vi "Scope_Fast_PID.vi"() -> ()   [LabVIEW 2013]
uses:
  <vilib>/userdefined/High Color/nirio_resource_hc.ctl
  FPGA/DataMode.ctl
  <vilib>/Analysis/4window.llb/windowTd.ctl
  Host/Scope/controls/power_spectrum_unit.ctl
  Host/Scope5782/Scope/controls/5782_trigger_type.ctl
  Host/Scope/controls/Data_calc_mode.ctl
  Host/Scope/controls/Data_display_mode.ctl
  Host/Scope/controls/Graph_references.ctl
  Host/Scope/controls/graph_controls.ctl
  Host/Scope/controls/Channel_select.ctl
  Host/Communication/response.ctl
  Host/Communication/driver_status.ctl
  Host/Communication/Driver/RemoteConnection/RemoteReferences.ctl
  Host/Scope5782/Config/FPGAref_5782.ctl
  Host/Communication/Driver/TcpServerDriver/TcpServerDriver.lvclass
  Host/Scope5782/Scope/controls/c_t_type.ctl
  Host/Scope/controls/ScopeMode.ctl
  FPGA/fpga_settings.ctl
  Host/Scope5782/Scope/controls/Memory block.ctl
  Host/Communication/global_stop.vi
  <vilib>/FPGAPlugInAG/PXIe-7975R/niLvFpga_Open_PXIe-7975R.vi
  <vilib>/rvi/interface/common/dynamic/niFpgaDynamicAddResources.vi
  <vilib>/rvi/interface/common/niFpgaWaitOnOcc.vi
  <vilib>/Utility/error.llb/Error Cluster From Error Code.vi
  <vilib>/rvi/errors/niLvFpgaAdjustHostInterfaceError.vi
  <vilib>/FPGAPlugInAG/Dynamic/niLvFpga_Close_Dynamic.vi
  <vilib>/rvi/interface/nirviOpenFPGA/nirviOpenFPGA.xnode
  FPGA Bitfiles/FPGAmain_5782_Fast_PID_eL07vsNfjYY.lvbitx
  <vilib>/rvi/interface/nirviReadWriteControl/nirviReadWriteControl.xnode
  <vilib>/rvi/FXPMathLib/FxpInterpret/XNode/nifxpmath_Interpret.xnode
  <vilib>/rvi/interface/nirviMethod/nirviMethod.xnode
  <vilib>/rvi/interface/nirviCloseFPGA/nirviCloseFPGA.xnode
  Host/Utilities/Ticker/Ticker.lvclass
  NiFpgaLv.dll
  <vilib>/rvi/interface/Simulation/niFpgaSimulationCallBeginRW.vi
  Host/Communication/Driver/RemoteConnection/RemoteConnection.lvclass
  <vilib>/FPGAPlugInAG/Dynamic/niLvFpga_WriteFifo_Dynamic.vi
  <vilib>/rvi/errors/niLvFpgaMergeErrorWithErrorCode.vi
  <vilib>/Analysis/NI_AALPro.lvlib
panel:
  in  "Acquire samples":u16
  in  "Trigger delay":u16
  in  "Feedback delay":u16
  in  "Beam/FF enabled":bool
  in  "Setpoint enabled":bool
  in  "show feedforward":bool
  in  "show beam":bool
  in  "show setpoint":bool
  in  "Feed forward":path
  in  "Beam":path
  in  "Setpoint":path
  in  "High speed transfer to host":bool=TRUE
  in  "Output enabled":bool=TRUE
  in  "ch1 DC offset":dbl caption="DC offset\nChannel 1"
  in  "ch0 DC offset":dbl caption="DC offset\nChannel 0"
  in  "Output delay delta":dbl(slide) scale=0.0..6.0
  in  "Output delay":dbl(slide) scale=0.0..6.0
  in  "Output mixer fequency [MHz]":dbl
  in  "Trigger":T1
  in  "Mode":T2
  in  "Mixer freq [MHz]":dbl
  in  "unwrap phase":bool
  in  "Kp AM":fxp<+/-,32,4> caption="Kp"
  in  "Kd/T AM":fxp<+/-,32,4> caption="Kd/T"
  in  "Ki*T AM":fxp<+/-,32,4> caption="Ki*T"
  in  "Feedback AM":bool caption="Feedback"
  in  "Kp":fxp<+/-,32,4>
  in  "Kd/T":fxp<+/-,32,4>
  in  "Ki*T":fxp<+/-,32,4>
  in  "Feedback":bool
  in  "c(t) AM":bool
  in  "c(t) phase":bool
  in  "b":fxp<+/-,16,2>
  in  "a":fxp<+/-,16,2>
  in  "Fequency [kHz]":dbl format="%#_8g"
  in  "#bins":i32=1 min=1 max=16
  in  "Unit":T3
  in  "Window":T4=1 items=["Rectangle"=0, "Hanning"=1, "Hamming"=2, "Blackman-Harris"=3, "Exact Blackman"=4, "Blackman"=5, "Flat Top"=6, "4 Term B-Harris "=7, "7 Term B-Harris"=8, "Low Sidelobe"=9, "Blackman Nuttall"=11, "Triangle"=30, "Bartlett-Hanning"=31, "Bohman"=32, "Parzen"=33, "Welch"=34, "Kaiser"=60, "Dolph-Chebyshev"=61, "Gaussian"=62]
  in  "Chart length":i32=400000
  in  "Trigmode":enum32{"Triggered", "Continuous"}(radio)
  in  "Refence for phase":T5
  in  "Graph_refs":T6
  out "Lower chart":dbl[][](graph)
  out "Upper chart":dbl[][](graph)
  out "Lower graph":i16[][](graph)
  in  "Buffer":T8
  in  "Display":T9
  in  "Ch1 Q":bool
  in  "Ch1 I":bool
  in  "Ch0 Q":bool
  in  "Ch0 I":bool
  in  "Ch1":bool
  in  "Ch0":bool
  out "stop 2":bool
  in  "Zoom freq X":bool
  in  "Zoom freq Y":bool
  in  "Zoom time Y":bool
  in  "Zoom time X":bool
  in  "Samples per 5782 record":i32
  in  "Phase offset (deg)":dbl
  in  "Fequency [MHz]":dbl format="%#_8g"
  out "freqdata":cluster{"f0":dbl, "df":dbl, "magnitude":dbl[]}[](graph)
  out "Upper graph":i16[][](graph)
  in  "Rumode":bool
  in  "Singleshot":bool
  out "error IO":errorcluster
  in  "stop":bool
  in  "resource name":T10="PXI1Slot18"
  out "Clocking Option Configured?":bool
  out "Configured?":bool
  # "Auto Zoom"
  # "5782"
  # "Delays"
  # "FFT"
  # "Auto Zoom"
  # "FPGA setup"
  # "V"
  # "V"
  # "ns"
  # "Output delay"
  # "ps"
  # "Output delay delta"
  # "Amplitude"
  # "Phase"
  # "Amplitude modulation"
  # "Simulated data"
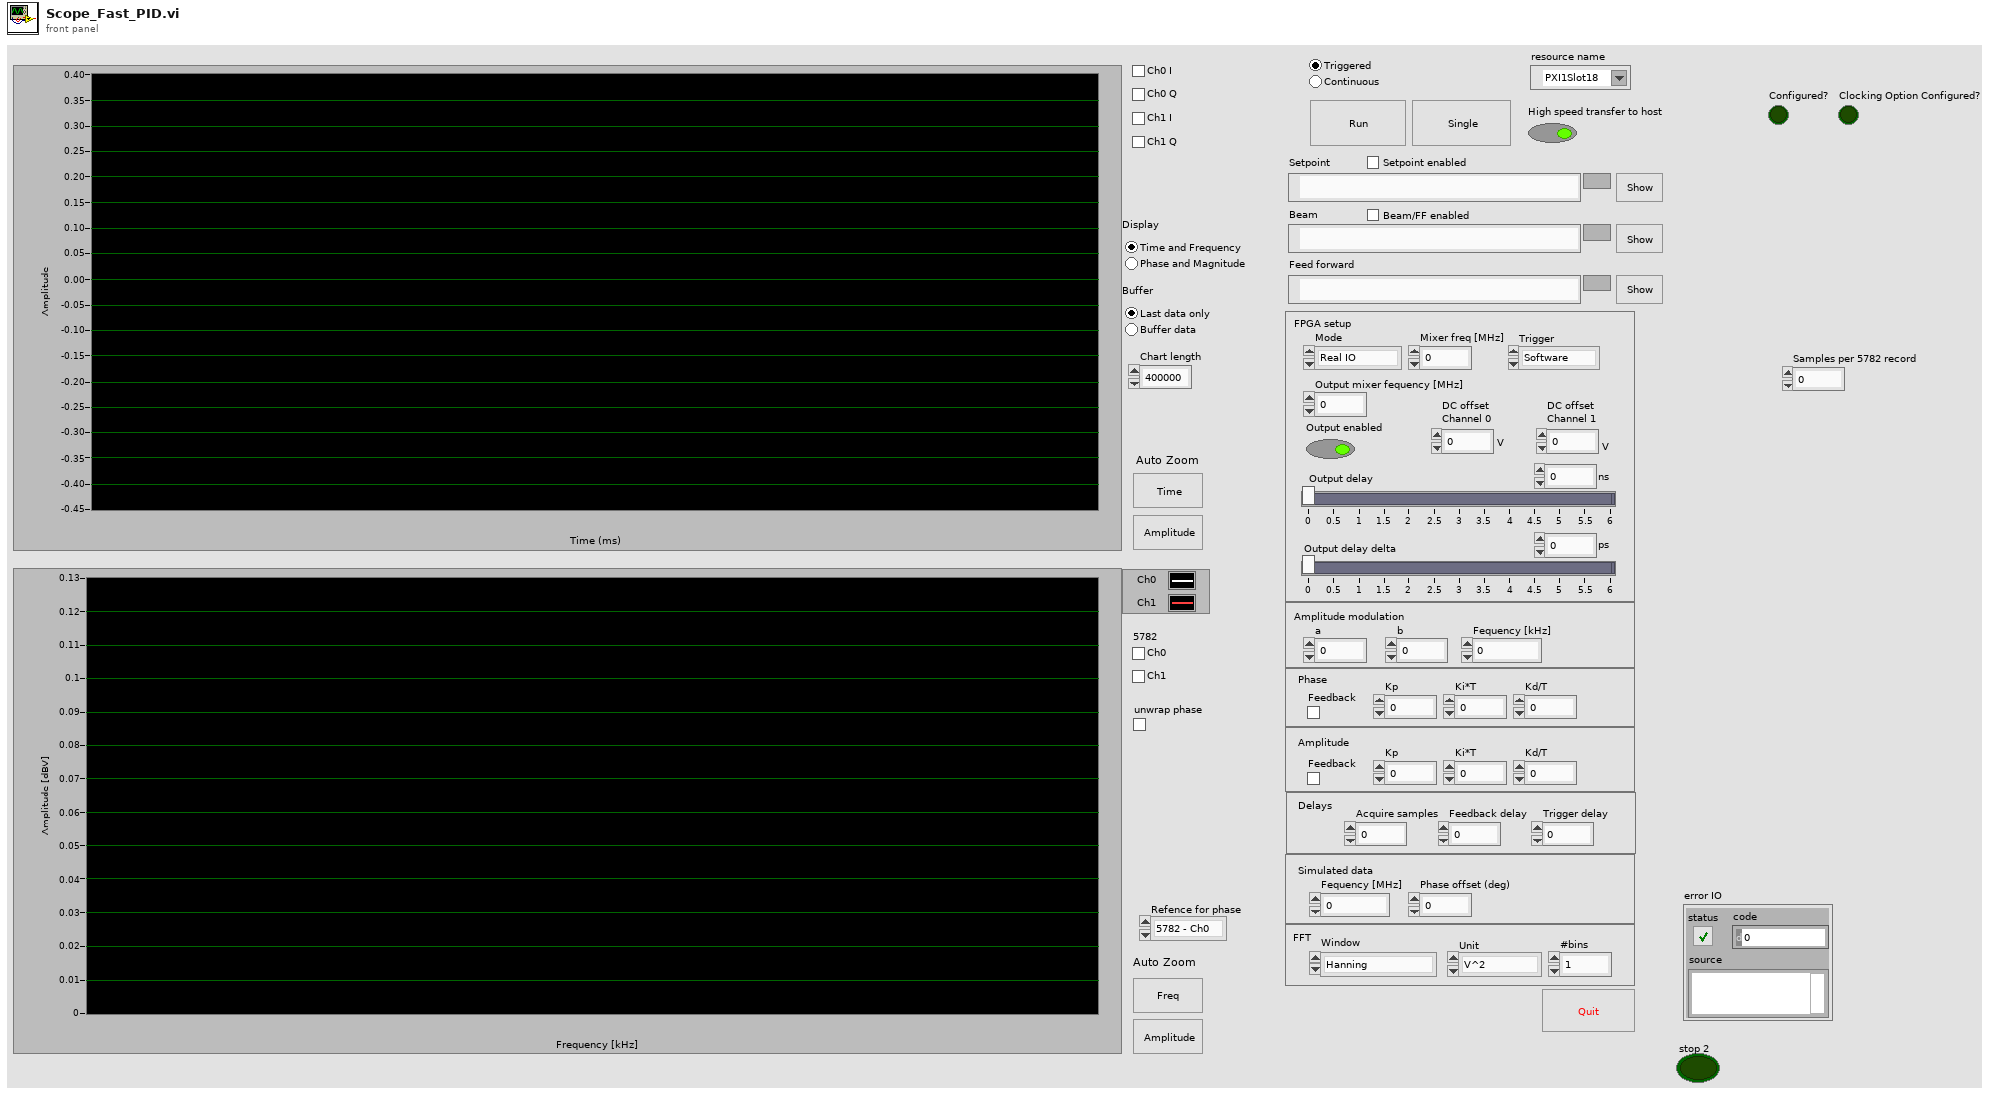
[diagram p1: front panel]
types:
  T1 = typedef "5782_trigger_type.ctl" = enum16{"Software", "Trigger input"}
  T2 = typedef "DataMode.ctl" = enum16{"Real IO", "Simulated"}
  T3 = typedef "power_spectrum_unit.ctl" = enum16{"V^2", "V", "dBV"}
  T4 = typedef "NI_AALPro.lvlib/windowTd.ctl" = u32
  T5 = typedef "Channel_select.ctl" = enum16{"5782 - Ch0", "5782 - Ch1"}
  T6 = typedef "Graph_references.ctl" = cluster{"upper":T7, "lower":T7, "Freq graph":refnum<vi>}
  T7 = typedef "graph_controls.ctl" = cluster{"Graph":refnum<vi>, "Time btn":refnum<vi>, "Amplitude btn":refnum<vi>, "Chart":refnum<vi>}
  T8 = typedef "Data_display_mode.ctl" = enum32{"Last data only", "Buffer data"}
  T9 = typedef "Data_calc_mode.ctl" = enum32{"Time and Frequency", "Phase and Magnitude"}
  T10 = typedef "nirio_resource_hc.ctl" = tag
  T11 = typedef "FPGAref_5782.ctl" = refnum<k20>
  T12 = typedef "RemoteConnection.lvclass/RemoteReferences.ctl" = cluster{"a":refnum<vi>, "b":refnum<vi>, "fm":refnum<vi>, "Output delay":refnum<vi>, "Output delay delta":refnum<vi>}
  T13 = typedef "response.ctl" = cluster{"driver status":T14, "Sender":string, "Type":i32, "Variant":variant}
  T14 = typedef "driver_status.ctl" = enum16{"Normal", "Startup", "Connection lost", "Reconnected", "Timeout", "Idle", "Busy"}
  T15 = enum8{"Internal Clock PLL Off", "Internal Clock PLL On (REF IN)", "External Clock (CLK_IN)", "Internal Clock PLL On (IoModSyncClk)"}
  T16 = typedef "message_queue.ctl" = refnum<queue>
  T17 = typedef "scope_params_5782.ctl" = cluster{"scope mode":T18, "ticker":refnum<class "Ticker.lvclass">, "samples per record":i32, "FPGA ref":T11, "data mode":T2, "5782 Trigger":T1, "Chart length":i32, "RemoteConnection":refnum<class "RemoteConnection.lvclass">, "last phase":dbl[], "Feedforward":T19}
  T18 = typedef "ScopeMode.ctl" = enum16{"Stopped", "Single", "Running", "Continuous"}
  T19 = typedef "Feedforward.ctl" = cluster{"Beam I":dbl[], "Beam Q":dbl[], "Feedforward I":dbl[], "Feedforward Q":dbl[], "Setpoint I":dbl[], "Setpoint Q":dbl[]}
  T20 = typedef "c_t_type.ctl" = enum16{"Phase", "AM", "Both", "None"}
  T21 = typedef "fpga_settings.ctl" = enum16{"Feedback Enable", "New FIR coeffs", "FIR shift", "Enable filter", "Set Downsample", "Downsample", "CIC Gain", "Record length", "Trigger samples", "Quiet time", "a_am", "b_am", "Use fixed delay", "fixed sin_fi", "fixed cos_fi", "Ki*Tau", "Kp", "Kd_Tau", "Fi_start", "Fi_delta", "DC_offs 0", "DC_offs 1", "DC_offs 2", "DC_offs 3", "Ki*Tau am", "Kp am", "Kd_Tau am", "Feedback AM", "Trigger delay", "Feedback delay", "Setpoint enable", "Beam enable", "Samples to acquire"}
  T22 = typedef "Memory block.ctl" = enum16{"Setpoint", "Beam"}
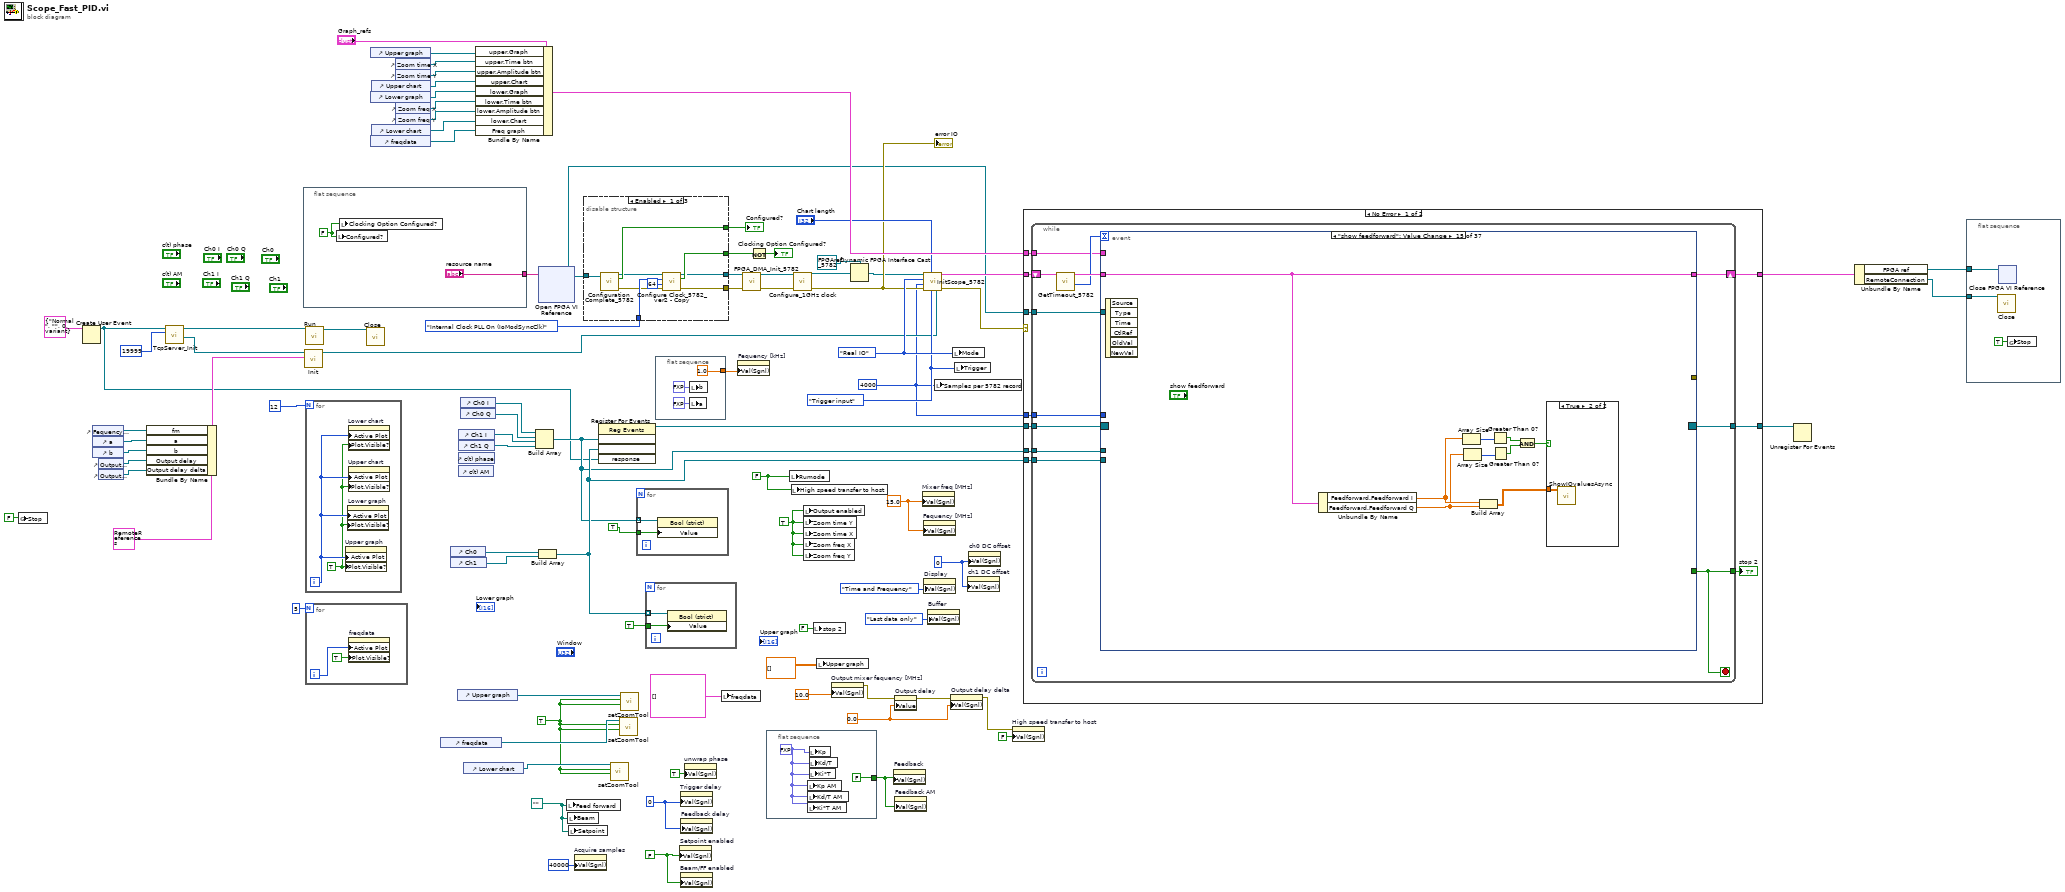
[diagram p0: block diagram]
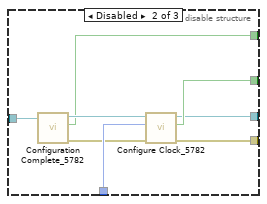
[diagram p2: hidden frame]
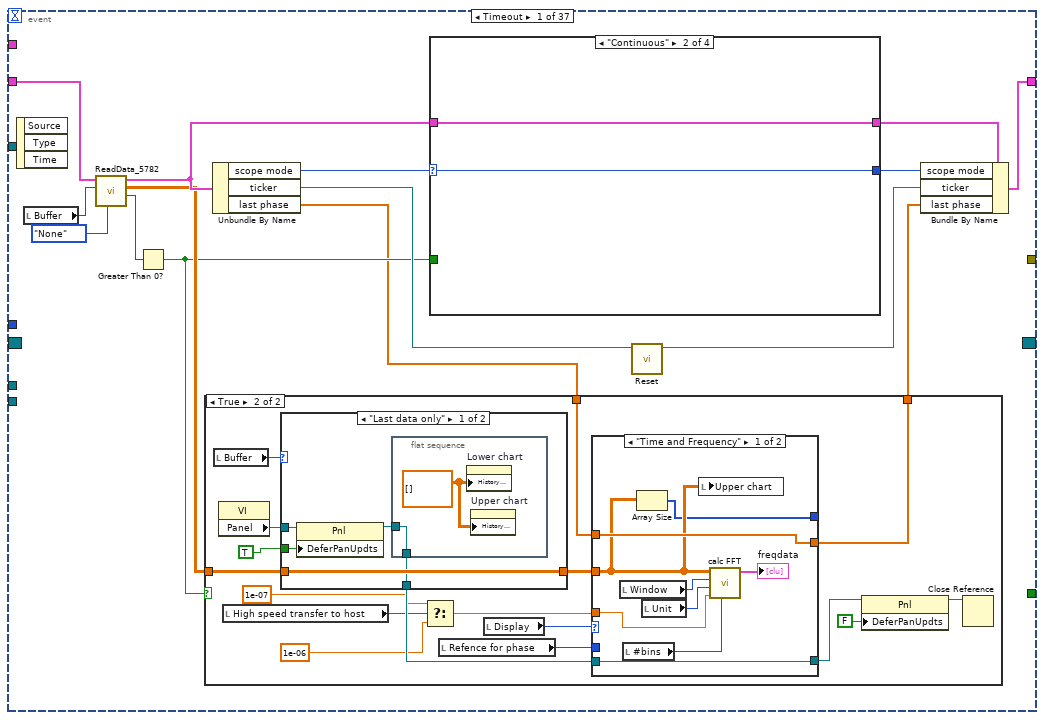
[diagram p4: hidden frame]
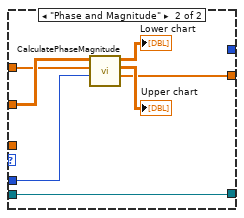
[diagram p7: hidden frame]
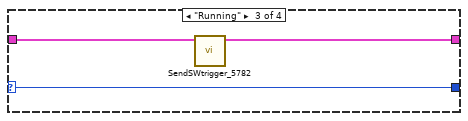
[diagram p9: hidden frame]
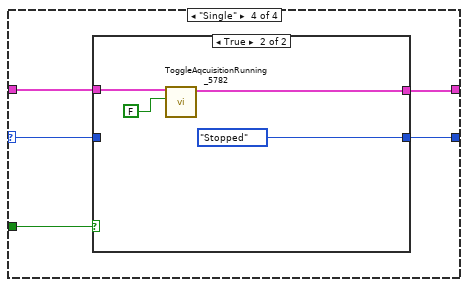
[diagram p10: hidden frame]
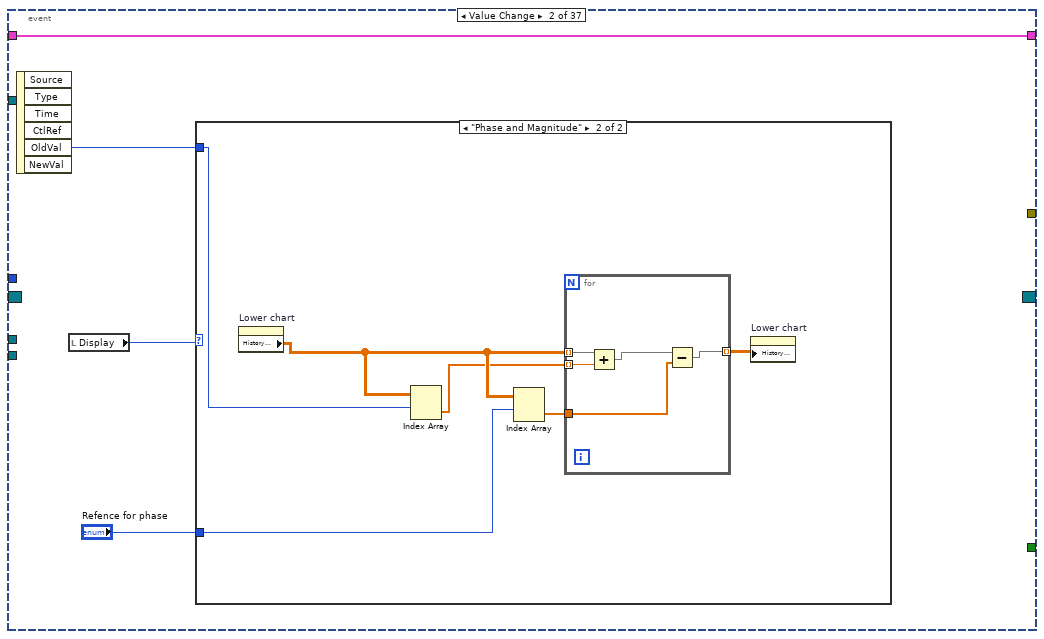
[diagram p12: hidden frame]
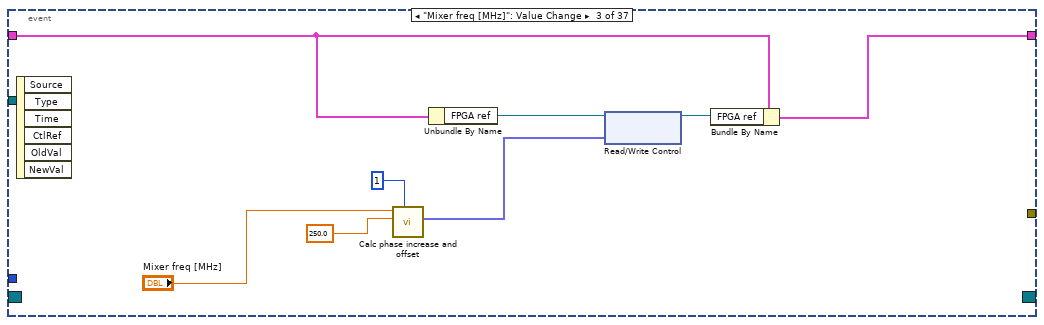
[diagram p14: hidden frame]
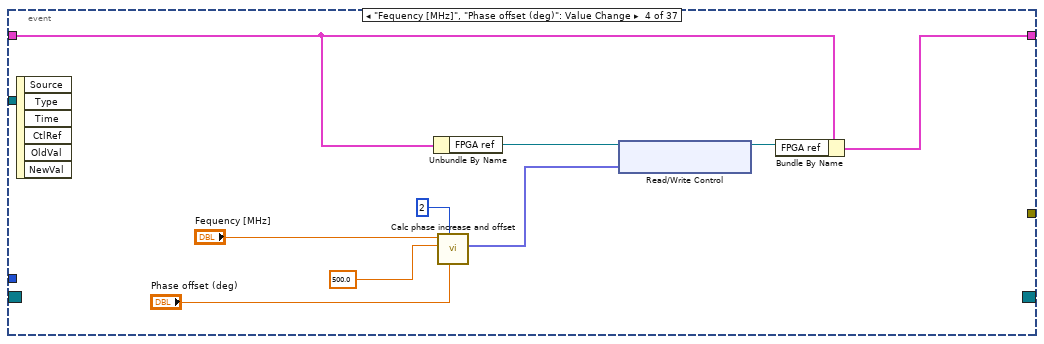
[diagram p15: hidden frame]
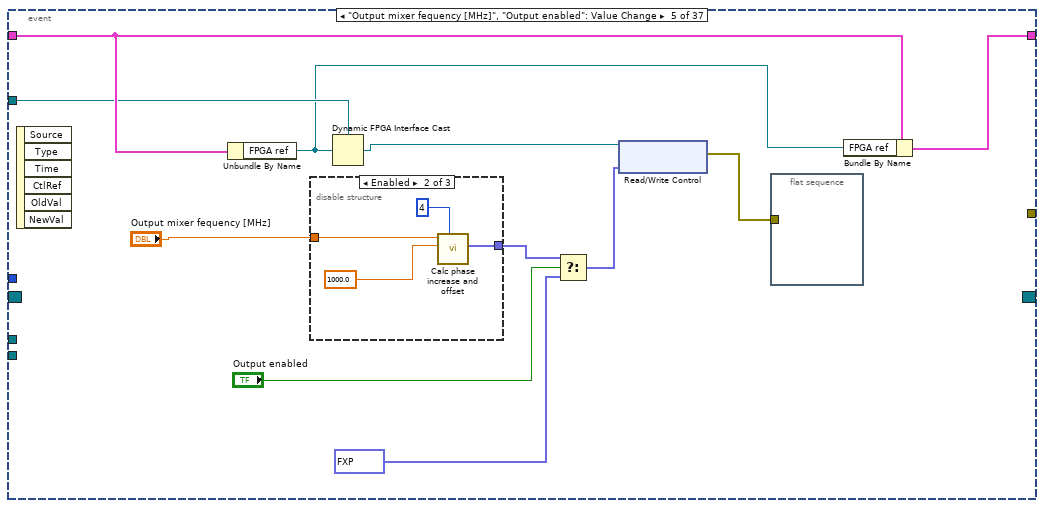
[diagram p16: hidden frame]
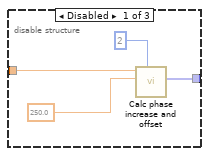
[diagram p17: hidden frame]
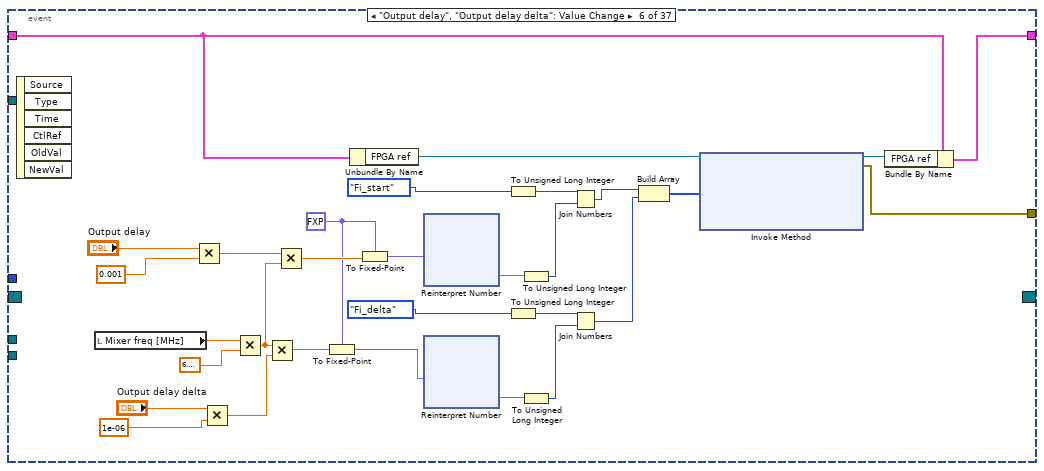
[diagram p19: hidden frame]
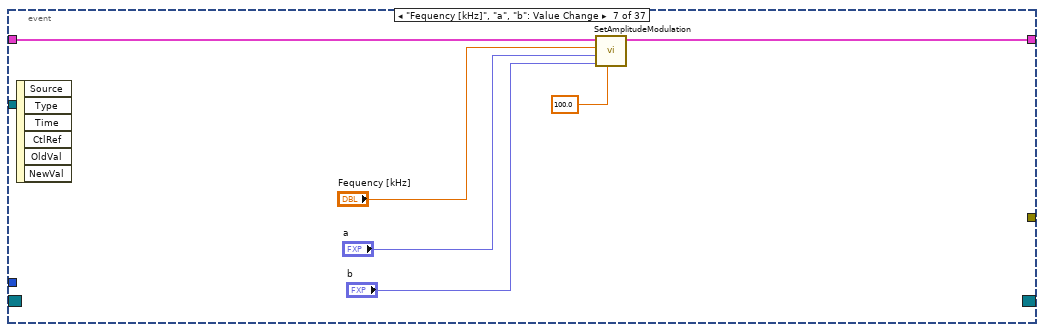
[diagram p20: hidden frame]
diagram:
  w2 = path "" ("Feed forward")
  w3 = FALSE ("Value (Signaling)")
  w4 = u16 0 ("Value (Signaling)")
  w40 = i16 0 ("Value (Signaling)")
  w41 = 0.0 ("Value (Signaling)")
  w63 = 5782_trigger_type."Trigger input" ("Trigger")
  w22 = TRUE ("Zoom  X")
  w15 = TRUE ("Rumode")
  w75 = DataMode."Real IO" ("Mode")
  w8 = 4000 ("Samples to aqcuire")
  w7 = FALSE ("Rumode")
  w85 = 15.0 ("Mixer requency [MHz]")
  n1 = global write "global_stop.vi" "Stop"(FALSE ("Stop")) -> ()
  n2 = Create User Event(user event datatype=T13 {"driver status"=enum."Normal", "Sender"="", "Type"=0, "Variant"=variant} ("response")) -> (user event=w28:refnum<user-event>)  [unwired: 1 in, 1 out]
  n3 = control-ref of="Fequency [kHz]"() -> (w30:refnum<vi>)
  n4 = control-ref of="a"() -> (w31:refnum<vi>)
  n5 = control-ref of="b"() -> (w29:refnum<vi>)
  n6 = control-ref of="Output delay"() -> (w18:refnum<vi>)
  n7 = control-ref of="Output delay delta"() -> (w17:refnum<vi>)
  n8 = Bundle By Name(cluster=T12 {"a"=refnum, "b"=refnum, "fm"=refnum, "Output delay"=refnum, "Output delay delta"=refnum} ("refs"), "fm"=w30, "a"=w31, "b"=w29, "Output delay"=w18, "Output delay delta"=w17) -> (w38:T12)
  n9 = call "TcpServer_Init.vi"("local port"=u16 19999, "response event"=w28) -> ("Message queue"=w36:T16, "TcpServerDriver"=w33:refnum<class "TcpServerDriver.lvclass">)  [unwired: 8 in]
  n10 = flat-sequence {
    tunnel: ["resource name"] -> w76
    frame #0 {
      w90 = FALSE ("Trigger Acquisition")
      n11 = local write "Configured?"(w90) -> ()
      n12 = local write "Clocking Option Configured?"(w90) -> ()
    }
  }
  n13 = call "Init.vi"("refs"=w38, "server queue"=w36) -> ("RemoteConnection"=w27:refnum<class "RemoteConnection.lvclass">)  [unwired: 9 in]
  n14 = for {
    N: 12 -> [_]
    i -> [w93]
    w92 = TRUE ("Plot.Visible")
    n15 = property on="Upper graph" class="WFGraph (strict)"("Active Plot"=w93, "Plot.Visible?"=w92) -> ()  [unwired: 2 in, 2 out]
    n16 = property on="Lower graph" class="WFGraph (strict)"("Active Plot"=w93, "Plot.Visible?"=w92) -> ()  [unwired: 2 in, 2 out]
    n17 = property on="Lower chart" class="WFChart (strict)"("Active Plot"=w93, "Plot.Visible?"=w92) -> ()  [unwired: 2 in, 2 out]
    n18 = property on="Upper chart" class="WFChart (strict)"("Active Plot"=w93, "Plot.Visible?"=w92) -> ()  [unwired: 2 in, 2 out]
  }
  n19 = for {
    N: 5 -> [_]
    i -> [w94]
    n20 = property on="freqdata" class="WFGraph (strict)"("Active Plot"=w94, "Plot.Visible?"=TRUE ("Plot.Visible")) -> ()  [unwired: 2 in, 2 out]
  }
  n21 = call-dynamic "Run.vi"("BaseDriver in"=w33) -> ("BaseDriver out"=w34:refnum<class "TcpServerDriver.lvclass">)  [unwired: 9 in, 1 out]
  n22 = call-dynamic "Close.vi"("BaseDriver in"=w34) -> ()  [unwired: 9 in, 2 out]
  n23 = control-ref of="Upper graph"() -> (w60:refnum<vi>)
  n24 = control-ref of="Lower graph"() -> (w56:refnum<vi>)
  n25 = control-ref of="freqdata"() -> (w52:refnum<vi>)
  n26 = control-ref of="Upper chart"() -> (w57:refnum<vi>)
  n27 = control-ref of="Lower chart"() -> (w53:refnum<vi>)
  n28 = control-ref of="Zoom time X"() -> (w59:refnum<vi>)
  n29 = control-ref of="Zoom time Y"() -> (w58:refnum<vi>)
  n30 = control-ref of="Zoom freq X"() -> (w55:refnum<vi>)
  n31 = control-ref of="Zoom freq Y"() -> (w54:refnum<vi>)
  n32 = control-ref of="freqdata"() -> (w65:refnum<vi>)
  n33 = control-ref of="Ch0"() -> (w72:refnum<vi>)
  n34 = control-ref of="Ch1"() -> (w73:refnum<vi>)
  n35 = control-ref of="Upper graph"() -> (w66:refnum<vi>)
  n36 = control-ref of="c(t) AM"() -> ()  [unwired: 1 out]
  n37 = control-ref of="Ch1 I"() -> (w70:refnum<vi>)
  n38 = control-ref of="Ch1 Q"() -> (w71:refnum<vi>)
  n39 = control-ref of="c(t) phase"() -> ()  [unwired: 1 out]
  n40 = control-ref of="Ch0 I"() -> (w68:refnum<vi>)
  n41 = control-ref of="Ch0 Q"() -> (w69:refnum<vi>)
  n42 = control-ref of="Lower chart"() -> (w23:refnum<vi>)
  n43 = Bundle By Name(cluster="Graph_refs", "upper.Graph"=w60, "upper.Time btn"=w59, "upper.Amplitude btn"=w58, "upper.Chart"=w57, "lower.Graph"=w56, "lower.Time btn"=w55, "lower.Amplitude btn"=w54, "lower.Chart"=w53, "Freq graph"=w52) -> (w51:T6)
  n44 = Build Array(w68, w69, w70, w71) -> (w67:refnum<vi>[])
  n45 = xnode "Open FPGA VI Reference"("resource name"=w76) -> ("FPGA VI Reference Out"=w9:refnum<k20>)  [unwired: 1 in, 1 out]
  n46 = Build Array(w72, w73) -> (w78:refnum<vi>[])
  n47 = local write "Feed forward"(w2) -> ()
  n48 = local write "Beam"(w2) -> ()
  n49 = local write "Setpoint"(w2) -> ()
  n50 = property on="Acquire samples" class="DigNum (strict)"("Val(Sgnl)"=u16 40000 ("Value (Signaling)")) -> ()  [unwired: 2 in, 2 out]
  n51 = disable-structure shown="Enabled" {
    disable-tunnel: [w104 w112 _] -> w47
    disable-tunnel: T15."Internal Clock PLL On (IoModSyncClk)" ("Clock Source") -> [w103 w111 _]
    disable-tunnel: [w101 w109 _] -> w46
    disable-tunnel: [w100 w106 w113] -> w13
    disable-tunnel: w9 -> [w96 w108 w113]
    disable-tunnel: [w99 w105 _] -> w44
    frame Enabled {
      n52 = call "Configuration Complete_5782.vi"("FPGA VI Reference in"=w96) -> ("error out"=w102:errorcluster, "Configured?"=w99:bool, "FPGA VI Reference out"=w98:refnum<k20>)  [unwired: 8 in]
      n53 = call "Configure Clock_5782_ver2 - Copy.vi"("error in"=w102, "User Data 1"=u8 64, "Clock Source"=w103, "FPGA VI Reference"=w98) -> ("error out"=w101:errorcluster, "Configuration Error"=w104:bool, "FPGA VI Reference out"=w100:refnum<k20>)  [unwired: 5 in]
    }
    frame Disabled {
      n54 = call "Configuration Complete_5782.vi"("FPGA VI Reference in"=w108) -> ("error out"=w110:errorcluster, "Configured?"=w105:bool, "FPGA VI Reference out"=w107:refnum<k20>)  [unwired: 8 in]
      n55 = call "Configure Clock_5782.vi"("error in"=w110, "Clock Source"=w111, "FPGA VI Reference in"=w107) -> ("error out"=w109:errorcluster, "Configuration Error"=w112:bool, "FPGA VI Reference Out"=w106:T11)  [unwired: 6 in]
    }
    frame Disabled {
    }
  }
  "Configured?" <- w44
  n56 = register-events(w67, w78, w28) -> (reference out=w82:refnum<event-registration>)  [unwired: 2 in, 1 out]
  n57 = call "setZoomTool.vi"("Zoom Y"=w22, "Zoom  X"=w22, "reference"=w23) -> ()  [unwired: 9 in]
  n58 = call "setZoomTool.vi"("Zoom Y"=w22, "Zoom  X"=w22, "reference"=w65) -> ()  [unwired: 9 in]
  n59 = call "setZoomTool.vi"("Zoom Y"=w22, "Zoom  X"=w22, "reference"=w66) -> ()  [unwired: 9 in]
  n60 = for {
    tunnel: w67 -> [w115] mode=indexing
    tunnel: TRUE ("Rumode") -> [w114]
    n61 = property class="Bool (strict)"(reference=w115, "Value"=w114) -> ()  [unwired: 1 in, 2 out]
  }
  n62 = for {
    tunnel: w78 -> [w117] mode=indexing
    tunnel: TRUE ("Rumode") -> [w116]
    n63 = property class="Bool (strict)"(reference=w117, "Value"=w116) -> ()  [unwired: 1 in, 2 out]
  }
  n64 = flat-sequence {
    tunnel: [1.0 ("Value (Signaling)")] -> w39
    frame #0 {
      n65 = local write "b"(fxp<+/-,16,2> 0.0 ("b")) -> ()
      n66 = local write "a"(fxp<+/-,16,2> 1.0 ("a")) -> ()
    }
  }
  n67 = property on="Setpoint enabled" class="Bool (strict)"("Val(Sgnl)"=w3) -> ()  [unwired: 2 in, 2 out]
  n68 = property on="Trigger delay" class="DigNum (strict)"("Val(Sgnl)"=w4) -> ()  [unwired: 2 in, 2 out]
  n69 = property on="Beam/FF enabled" class="Bool (strict)"("Val(Sgnl)"=w3) -> ()  [unwired: 2 in, 2 out]
  n70 = property on="Feedback delay" class="DigNum (strict)"("Val(Sgnl)"=w4) -> ()  [unwired: 2 in, 2 out]
  n71 = property on="unwrap phase" class="Bool (strict)"("Val(Sgnl)"=TRUE ("Value (Signaling)")) -> ()  [unwired: 2 in, 2 out]
  n72 = local write "freqdata"(cluster{"f0":dbl, "df":dbl, "magnitude":dbl[]}[] [] ("freqdata")) -> ()
  n73 = property on="Fequency [kHz]" class="DigNum (strict)"("Val(Sgnl)"=w39) -> ()  [unwired: 2 in, 2 out]
  n74 = call "FPGA_DMA_Init_5782.vi"("error in (no error)"=w46, "FPGA VI Reference"=w13) -> ("error out"=w21:errorcluster, "FPGA VI Out"=w14:refnum<k20>)  [unwired: 7 in, 1 out]
  n75 = Not(x=w47) -> (.not. x?=→"Clocking Option Configured?":bool)
  n76 = flat-sequence {
    tunnel: [FALSE] -> w19
    frame #0 {
      w121 = fxp<+/-,32,4> 0.0 ("Kp")
      n77 = local write "Kp AM"(w121) -> ()
      n78 = local write "Kd/T AM"(w121) -> ()
      n79 = local write "Ki*T AM"(w121) -> ()
      n80 = local write "Kp"(w121) -> ()
      n81 = local write "Kd/T"(w121) -> ()
      n82 = local write "Ki*T"(w121) -> ()
    }
  }
  n83 = local write "Rumode"(w7) -> ()
  n84 = local write "High speed transfer to host"(w7) -> ()
  n85 = call "Configure_1GHz clock.vi"("error in"=w21, "FPGA SPI config ref"=w14) -> ("error out"=w20:errorcluster, "FPGA SPI config out"=w11:refnum<k20>)  [unwired: 8 in]
  "error IO" <- w20
  n86 = local write "Output enabled"(w15) -> ()
  n87 = local write "Zoom time Y"(w15) -> ()
  n88 = local write "Zoom time X"(w15) -> ()
  n89 = local write "Zoom freq X"(w15) -> ()
  n90 = local write "Zoom freq Y"(w15) -> ()
  n91 = local write "stop 2"(FALSE ("stop 2")) -> ()
  n92 = local write "Upper graph"(dbl[][] [] ("Timedata")) -> ()
  n93 = property on="Output mixer fequency [MHz]" class="DigNum (strict)"("Val(Sgnl)"=10.0 ("Mixer requency [MHz]")) -> (error out=w42:errorcluster)  [unwired: 2 in, 1 out]
  n94 = Dynamic FPGA Interface Cast(Session In=T11 refnum ("FPGA ref"), Type=w11) -> (Session Out=w10:T11)
  n95 = property on="Feedback" class="Bool (strict)"("Val(Sgnl)"=w19) -> ()  [unwired: 2 in, 2 out]
  n96 = property on="Output delay" class="Slide (strict)"(error in=w42, "Value"=w41) -> (error out=w43:errorcluster)  [unwired: 1 in, 1 out]
  n97 = property on="Feedback AM" class="Bool (strict)"("Val(Sgnl)"=w19) -> ()  [unwired: 2 in, 2 out]
  n98 = property on="Mixer freq [MHz]" class="DigNum (strict)"("Val(Sgnl)"=w85) -> ()  [unwired: 2 in, 2 out]
  n99 = property on="Fequency [MHz]" class="DigNum (strict)"("Val(Sgnl)"=w85) -> ()  [unwired: 2 in, 2 out]
  n100 = call "InitScope_5782.vi"("RemoteConnection"=w27, "Trigger"=w63, "Chart length"="Chart length", "error in"=w20, "Samples Per Trigger"=w8, "data mode"=w75, "FPGA ref"=w10) -> ("error out"=w24:errorcluster, "scope params"=w89:T17)  [unwired: 3 in]
  n101 = property on="Display" class="RadioBtnsControl (strict)"("Val(Sgnl)"=Data_calc_mode."Time and Frequency" ("Value (Signaling)")) -> ()  [unwired: 2 in, 2 out]
  n102 = property on="Buffer" class="RadioBtnsControl (strict)"("Val(Sgnl)"=enum32{"Last data only", "Buffer data"}."Last data only" ("Value (Signaling)")) -> ()  [unwired: 2 in, 2 out]
  n103 = local write "Samples per 5782 record"(w8) -> ()
  n104 = property on="Output delay delta" class="Slide (strict)"(error in=w43, "Val(Sgnl)"=w41) -> (error out=w6:errorcluster)  [unwired: 1 in, 1 out]
  n105 = local write "Mode"(w75) -> ()
  n106 = local write "Trigger"(w63) -> ()
  n107 = property on="ch1 DC offset" class="DigNum (strict)"("Val(Sgnl)"=w40) -> ()  [unwired: 2 in, 2 out]
  n108 = property on="ch0 DC offset" class="DigNum (strict)"("Val(Sgnl)"=w40) -> ()  [unwired: 2 in, 2 out]
  n109 = property on="High speed transfer to host" class="Bool (strict)"(error in=w6, "Val(Sgnl)"=FALSE ("Value (Signaling)")) -> ()  [unwired: 1 in, 2 out]
  n110 = case shown="No Error" w24 {
    tunnel: w89 -> [w132 w661]
    tunnel: [w131 w661] -> w64
    tunnel: w82 -> [w130 w660]
    tunnel: [w129 w660] -> w81
    tunnel: w67 -> [w128 _]
    tunnel: w78 -> [w127 _]
    tunnel: w51 -> [w125 _]
    tunnel: w9 -> [w124 _]
    tunnel: w8 -> [w123 _]
    frame No Error {
      n111 = while {
        shift-right: [w144] -> w131
        shift-left: w132 -> [w143]
        tunnel: w130 -> [w140]
        tunnel: [w139] -> w129
        tunnel: w128 -> [w138]
        tunnel: w127 -> [w137]
        tunnel: [w136] -> w126
        tunnel: w125 -> [w135]
        tunnel: w124 -> [w134]
        tunnel: w123 -> [w133]
        stop <- w136 stop-if-true
        n112 = call "GetTimeout_5782.vi"("scope in"=w143) -> ("Time left"=w141:i32, "scope out"=w142:T17)  [unwired: 9 in]
        n113 = event shown="[14] \"show feedforward\": Value Change" {
          selector: w140 -> [_ _ _ _ _ _ _ _ _ _ _ _ _ _ _ _ _ _ _ _ _ _ _ _ _ _ _ _ _ _ _ _ _ _ _ _ _]
          dyn-events: [_ _ _ _ _ _ _ _ _ _ _ _ _ _ _ _ _ _ _ _ _ _ _ _ _ _ _ _ _ _ _ _ _ _ _ _ _] -> w139
          timeout: w141 -> [_ _ _ _ _ _ _ _ _ _ _ _ _ _ _ _ _ _ _ _ _ _ _ _ _ _ _ _ _ _ _ _ _ _ _ _ _]
          tunnel: [_ _ _ _ _ _ _ _ _ _ _ _ _ _ _ _ _ _ _ _ _ _ _ _ _ _ _ _ "stop" _ _ _ _ _ _ _ _] -> w136
          tunnel: w142 -> [w154 w224 w242 w248 w263 w299 w307 w335 w363 w377 w391 w399 w400 w410 w420 w443 w453 w463 w467 w471 w486 w495 w505 w513 w538 w549 w562 w567 w570 w577 w587 w592 w598 w605 w614 w633 w652]
          tunnel: [w157 w224 w240 w247 w262 w298 w306 w334 w362 w376 w390 w398 w400 w410 w420 w442 w452 w462 w466 w470 w485 w494 w502 w510 w538 w549 w562 w566 w570 w577 w587 w592 w598 w605 w611 w630 w649] -> w144
          tunnel: w138 -> [_ _ _ _ _ _ _ _ _ _ _ _ _ _ _ _ _ _ _ _ _ _ _ _ w537 _ _ _ _ _ _ _ _ _ _ _ _]
          tunnel: w137 -> [_ _ _ _ _ _ _ _ _ _ _ _ _ _ _ _ _ _ _ _ _ _ _ _ _ w547 _ _ _ _ _ _ _ _ _ _ _]
          tunnel: w135 -> [_ _ _ _ _ _ _ _ _ _ _ _ _ _ _ _ _ _ _ _ _ _ _ _ _ _ _ _ _ _ _ _ _ w602 _ _ _]
          tunnel: w134 -> [_ _ _ _ w254 _ _ _ _ _ _ _ _ _ _ _ _ _ _ _ w488 _ _ _ _ _ _ _ _ _ _ _ _ _ w608 w627 w646]
          tunnel: w133 -> [_ _ _ _ _ _ _ _ _ _ _ _ _ _ _ _ _ _ _ _ w491 _ _ _ _ _ _ _ _ _ _ _ _ _ _ _ _]
          tunnel: [_ _ _ _ _ w272 _ _ _ _ _ _ _ _ _ _ _ _ _ _ _ _ _ _ _ _ _ _ _ _ _ _ _ _ _ _ _] -> _
          event Timeout {
            n114 = event-data() -> ()  [unwired: 1 in, 3 out]
            n115 = local read "Buffer"() -> (w148:T8)
            n116 = call "ReadData_5782.vi"("c(t)"=c_t_type."None", "Buffer mode"=w148, "scope params"=w154) -> ("Num elements"=w150:i32, "data"=w151:dbl[][], "scope params out"=w153:T17)  [unwired: 6 in]
            n117 = Greater Than 0?(x=w150) -> (x > 0?=w149:bool)
            n118 = Unbundle By Name(w153) -> ("scope mode"=w156:T18, "ticker"=w159:refnum<class "Ticker.lvclass">, "last phase"=w147:dbl[])
            n119 = case shown="True" w149 {
              tunnel: w151 -> [_ w174]
              tunnel: w147 -> [w160 w166]
              tunnel: [w160 w165] -> w146
              frame False {
              }
              frame True {
                n120 = local read "Buffer"() -> (w176:T8)
                n121 = property class="VI"() -> ("Panel"=w169:refnum<vi>)  [unwired: 2 in, 2 out]
                n122 = local read "High speed transfer to host"() -> (w164:bool)
                n123 = case shown="\"Last data only\"" w176 {
                  tunnel: w174 -> [w182 w186]
                  tunnel: [w182 w186] -> w175
                  tunnel: w169 -> [w181 w185]
                  tunnel: TRUE ("Defer Panel Updates") -> [w179 _]
                  tunnel: [w178 w185] -> w167
                  frame "Last data only" {
                    n124 = property class="Pnl"(reference=w181, "DeferPanUpdts"=w179) -> (reference out=w180:refnum<vi>)  [unwired: 1 in, 1 out]
                    n125 = flat-sequence {
                      tunnel: w180 -> [w183]
                      tunnel: [w183] -> w178
                      frame #0 {
                        w184 = dbl[][] [] ("History Data")
                        n126 = property on="Lower chart" class="WFChart (strict)"("History Data"=w184) -> ()  [unwired: 2 in, 2 out]
                        n127 = property on="Upper chart" class="WFChart (strict)"("History Data"=w184) -> ()  [unwired: 2 in, 2 out]
                      }
                    }
                  }
                  frame "Buffer data" {
                  }
                }
                n128 = Select(t=1e-07 ("dt"), s=w164, f=1e-06 ("dt")) -> (s? t:f=w161:dbl)
                n129 = local read "Refence for phase"() -> (w173:T5)
                n130 = local read "Display"() -> (w177:T9)
                n131 = case shown="\"Time and Frequency\"" w177 {
                  tunnel: w175 -> [w188 w202]
                  tunnel: w173 -> [_ w199]
                  tunnel: [w192 w198] -> w171
                  tunnel: w167 -> [w192 w198]
                  tunnel: w166 -> [w190 w197]
                  tunnel: [w190 w196] -> w165
                  tunnel: w161 -> [w189 _]
                  tunnel: [w187 _] -> _
                  frame "Time and Frequency" {
                    n132 = local read "Window"() -> (w193:T4)
                    n133 = local read "#bins"() -> (w191:i32)
                    n134 = Array Size(array=w188) -> (size(s)=w187:i32[])
                    n135 = local read "Unit"() -> (w194:T3)
                    n136 = local write "Upper chart"(w188) -> ()
                    n137 = call "calc FFT.vi"("#bins"=w191, "dt"=w189, "Unit"=w194, "Window"=w193, "data"=w188) -> ("Power Spectrum / PSD"=→"freqdata":cluster{"f0":dbl, "df":dbl, "magnitude":dbl[]}[])  [unwired: 6 in]
                  }
                  frame "Phase and Magnitude" {
                    n138 = call "CalculatePhaseMagnitude.vi"("phase reference channel"=w199, "previous phase"=w197, "data"=w202) -> ("last phase"=w196:dbl[], "Magnitude"=→"Upper chart":dbl[][], "Phase"=→"Lower chart":dbl[][])  [unwired: 6 in]
                  }
                }
                n139 = property class="Pnl"(reference=w171, "DeferPanUpdts"=FALSE ("Defer Panel Updates")) -> (reference out=w170:refnum<vi>)  [unwired: 1 in, 1 out]
                n140 = Close Reference(reference=w170) -> ()  [unwired: 1 in, 1 out]
              }
            }
            n141 = case shown="\"Continuous\"" w156 {
              selector: w156 -> [w204 w206 w209 w210]
              tunnel: [w204 w206 w209 w214] -> w155
              tunnel: w153 -> [w203 w205 w208 w212]
              tunnel: [w203 w205 w207 w211] -> w152
              tunnel: w149 -> [_ _ _ w213]
              frame "Stopped" {
              }
              frame "Continuous" {
              }
              frame "Running" {
                n142 = call "SendSWtrigger_5782.vi"("scope in"=w208) -> ("scope out"=w207:T17)  [unwired: 9 in, 1 out]
              }
              frame "Single" {
                n143 = case shown="True" w213 {
                  tunnel: [w215 ScopeMode."Stopped" ("scope mode")] -> w214
                  tunnel: w212 -> [w216 w219]
                  tunnel: [w216 w218] -> w211
                  tunnel: w210 -> [w215 _]
                  frame False {
                  }
                  frame True {
                    n144 = call "ToggleAqcuisitionRunning_5782.vi"("Acquisition running"=FALSE, "scope in"=w219) -> ("scope out"=w218:T17)  [unwired: 8 in, 1 out]
                  }
                }
              }
            }
            n145 = call "Reset.vi"("Ticker in"=w159) -> ("Ticker out"=w158:refnum<class "Ticker.lvclass">)  [unwired: 9 in, 1 out]
            n146 = Bundle By Name(cluster=w152, "scope mode"=w155, "ticker"=w158, "last phase"=w146) -> (w157:T17)
          }
          event Value Change {
            n147 = event-data() -> ("OldVal"=w221:T5)  [unwired: 1 in, 5 out]
            n148 = local read "Display"() -> (w222:T9)
            n149 = case shown="\"Phase and Magnitude\"" w222 {
              tunnel: "Refence for phase" -> [_ w229]
              tunnel: w221 -> [_ w227]
              frame "Time and Frequency", Default {
              }
              frame "Phase and Magnitude" {
                n150 = property on="Lower chart" class="WFChart (strict)"() -> ("History Data"=w228:dbl[][])  [unwired: 2 in, 2 out]
                n151 = Index Array(array=w228, index (row)=w227) -> (element=w226:dbl[])  [unwired: 1 in]
                n152 = Index Array(array=w228, index (row)=w229) -> (element=w230:dbl[])  [unwired: 1 in]
                n153 = for {
                  tunnel: w228 -> [w233] mode=indexing
                  tunnel: w230 -> [w235]
                  tunnel: [w234] -> w225 mode=indexing
                  tunnel: w226 -> [w232] mode=indexing
                  n154 = Add(x=w233, y=w232) -> (x+y=w231:dbl[])
                  n155 = Subtract(x=w231, y=w235) -> (x-y=w234:dbl[])
                }
                n156 = property on="Lower chart" class="WFChart (strict)"("History Data"=w225) -> ()  [unwired: 2 in, 2 out]
              }
            }
          }
          event "Mixer freq [MHz]": Value Change {
            n157 = event-data() -> ()  [unwired: 1 in, 6 out]
            n158 = call "Calc phase increase and offset.vi"("# of DDS"=1, "fclk (MHz)"=250.0 ("fclk (800MHz)"), "f_generated (MHz)"="Mixer freq [MHz]") -> ("Phase out"=w236:fxp<+,64,64>[])  [unwired: 6 in, 2 out]
            n159 = Unbundle By Name(w242) -> ("FPGA ref"=w243:T11)
            n160 = xnode "Read/Write Control"("FPGA VI Reference In"=w243, "Phase 5782"=w236) -> ("FPGA VI Reference Out"=w241:T11)  [unwired: 1 in, 1 out]
            n161 = Bundle By Name(cluster=w242, "FPGA ref"=w241) -> (w240:T17)
          }
          event "Fequency [MHz]", "Phase offset (deg)": Value Change {
            n162 = event-data() -> ()  [unwired: 1 in, 6 out]
            n163 = Unbundle By Name(w248) -> ("FPGA ref"=w250:T11)
            n164 = call "Calc phase increase and offset.vi"("Phase offset (deg)"="Phase offset (deg)", "# of DDS"=2, "fclk (MHz)"=500.0 ("fclk (800MHz)"), "f_generated (MHz)"="Fequency [MHz]") -> ("Phase out"=w244:fxp<+,64,64>[])  [unwired: 5 in, 2 out]
            n165 = xnode "Read/Write Control"("FPGA VI Reference In"=w250, "Simulated phase 5782"=w244) -> ("FPGA VI Reference Out"=w249:T11)  [unwired: 1 in, 1 out]
            n166 = Bundle By Name(cluster=w248, "FPGA ref"=w249) -> (w247:T17)
          }
          event "Output mixer fequency [MHz]", "Output enabled": Value Change {
            n167 = event-data() -> ()  [unwired: 1 in, 6 out]
            n168 = Unbundle By Name(w263) -> ("FPGA ref"=w253:T11)
            n169 = disable-structure shown="Enabled" {
              disable-tunnel: [w265 w269 _] -> w257
              disable-tunnel: "Output mixer fequency [MHz]" -> [w264 w268 _]
              frame Disabled {
                n170 = call "Calc phase increase and offset.vi"("# of DDS"=2, "fclk (MHz)"=250.0 ("fclk (800MHz)"), "f_generated (MHz)"=w264) -> ("Phase out"=w265:fxp<+,64,64>[])  [unwired: 6 in, 2 out]
              }
              frame Enabled {
                n171 = call "Calc phase increase and offset.vi"("# of DDS"=4, "fclk (MHz)"=1000.0 ("fclk (800MHz)"), "f_generated (MHz)"=w268) -> ("Phase out"=w269:fxp<+,64,64>[])  [unwired: 6 in, 2 out]
              }
              frame Disabled {
              }
            }
            n172 = Dynamic FPGA Interface Cast(Session In=w254, Type=w253) -> (Session Out=w255:refnum<k20>)
            n173 = Select(t=w257, s="Output enabled", f=fxp<+,64,64>[] [0.0, 0.0, 0.0, 0.0]) -> (s? t:f=w256:fxp<+,64,64>[])
            n174 = xnode "Read/Write Control"("FPGA VI Reference In"=w255, "Phase output"=w256) -> ("error out"=w260:errorcluster)  [unwired: 1 in, 1 out]
            n175 = flat-sequence {
              tunnel: w260 -> [_]
              frame #0 {
              }
            }
            n176 = Bundle By Name(cluster=w263, "FPGA ref"=w253) -> (w262:T17)
          }
          event "Output delay", "Output delay delta": Value Change {
            w278 = fxp<+/-,32,4> 0.0 ("x")
            n177 = event-data() -> ()  [unwired: 1 in, 6 out]
            n178 = local read "Mixer freq [MHz]"() -> (w293:dbl)
            n179 = Multiply(x="Output delay", y=0.001) -> (x*y=w294:dbl)
            n180 = Multiply(x="Output delay delta", y=1e-06) -> (x*y=w296:dbl)
            n181 = Multiply(x=w293, y=6.283185307179586) -> (x*y=w291:dbl)
            n182 = Multiply(x=w291, y=w296) -> (x*y=w279:dbl)
            n183 = Multiply(x=w294, y=w291) -> (x*y=w281:dbl)
            n184 = To Fixed-Point(fixed-point type=w278, number=w279) -> (fixed-point=w277:fxp<+/-,32,4>)
            n185 = Unbundle By Name(w299) -> ("FPGA ref"=w274:T11)
            n186 = To Fixed-Point(fixed-point type=w278, number=w281) -> (fixed-point=w280:fxp<+/-,32,4>)
            n187 = xnode "Reinterpret Number"("x"=w280) -> ("y"=w287:fxp<+,32,32>)
            n188 = xnode "Reinterpret Number"("x"=w277) -> ("y"=w286:fxp<+,32,32>)
            n189 = To Unsigned Long Integer(number=fpga_settings."Fi_start" ("FPGA Setting")) -> (unsigned 32bit integer=w290:u32)
            n190 = To Unsigned Long Integer(number=fpga_settings."Fi_delta" ("FPGA Setting")) -> (unsigned 32bit integer=w283:u32)
            n191 = To Unsigned Long Integer(number=w287) -> (unsigned 32bit integer=w289:u32)
            n192 = To Unsigned Long Integer(number=w286) -> (unsigned 32bit integer=w284:u32)
            n193 = Join Numbers(hi=w290, lo=w289) -> ((hi.lo)=w275:u64)
            n194 = Join Numbers(hi=w283, lo=w284) -> ((hi.lo)=w276:u64)
            n195 = Build Array(w275, w276) -> (w282:u64[])
            n196 = xnode "Invoke Method"("FPGA VI Reference In"=w274, "Data"=w282) -> ("FPGA VI Reference Out"=w273:T11, "error out"=w272:errorcluster)  [unwired: 2 in, 1 out]
            n197 = Bundle By Name(cluster=w299, "FPGA ref"=w273) -> (w298:T17)
          }
          event "Fequency [kHz]", "a", "b": Value Change {
            n198 = event-data() -> ()  [unwired: 1 in, 6 out]
            n199 = call "SetAmplitudeModulation.vi"("fclk (MHz)"=100.0, "b_am"="b", "a_am"="a", "Am freq [kHz]"="Fequency [kHz]", "scope in"=w307) -> ("scope out"=w306:T17)  [unwired: 6 in]
          }
          event "Feedback": Value Change {
            n200 = event-data() -> ()  [unwired: 1 in, 6 out]
            n201 = xnode "Reinterpret Number"("x"="Kd/T") -> ("y"=w321:fxp<+,32,32>)
            n202 = xnode "Reinterpret Number"("x"="Ki*T") -> ("y"=w318:fxp<+,32,32>)
            n203 = xnode "Reinterpret Number"("x"="Kp") -> ("y"=w325:fxp<+,32,32>)
            n204 = Unbundle By Name(w335) -> ("FPGA ref"=w333:T11)
            n205 = To Unsigned Long Integer(number=fpga_settings."Kd_Tau" ("FPGA Setting")) -> (unsigned 32bit integer=w319:u32)
            n206 = To Unsigned Long Integer(number=fpga_settings."Ki*Tau" ("FPGA Setting")) -> (unsigned 32bit integer=w315:u32)
            n207 = To Unsigned Long Integer(number=fpga_settings."Kp" ("FPGA Setting")) -> (unsigned 32bit integer=w322:u32)
            n208 = To Unsigned Long Integer(number=w318) -> (unsigned 32bit integer=w314:u32)
            n209 = To Unsigned Long Integer(number=w321) -> (unsigned 32bit integer=w320:u32)
            n210 = Boolean To (0,1)(Boolean="Feedback") -> (0, 1=w330:i16)
            n211 = To Unsigned Long Integer(number=w325) -> (unsigned 32bit integer=w324:u32)
            n212 = To Unsigned Long Integer(number=w330) -> (unsigned 32bit integer=w327:u32)
            n213 = Join Numbers(hi=w315, lo=w314) -> ((hi.lo)=w313:u64)
            n214 = Join Numbers(hi=w319, lo=w320) -> ((hi.lo)=w312:u64)
            n215 = Join Numbers(hi=w322, lo=w324) -> ((hi.lo)=w332:u64)
            n216 = Join Numbers(hi=fpga_settings."Feedback Enable" ("FPGA Setting"), lo=w327) -> ((hi.lo)=w328:u64)
            n217 = Build Array(w328, w313, w312, w332) -> (w331:u64[])
            n218 = xnode "Invoke Method"("FPGA VI Reference In"=w333, "Data"=w331) -> ("FPGA VI Reference Out"=w308:T11)  [unwired: 2 in, 2 out]
            n219 = Bundle By Name(cluster=w335, "FPGA ref"=w308) -> (w334:T17)
          }
          event "Feedback AM": Value Change {
            n220 = event-data() -> ()  [unwired: 1 in, 6 out]
            n221 = xnode "Reinterpret Number"("x"="Kd/T AM") -> ("y"=w350:fxp<+,32,32>)
            n222 = xnode "Reinterpret Number"("x"="Ki*T AM") -> ("y"=w347:fxp<+,32,32>)
            n223 = xnode "Reinterpret Number"("x"="Kp AM") -> ("y"=w354:fxp<+,32,32>)
            n224 = Unbundle By Name(w363) -> ("FPGA ref"=w361:T11)
            n225 = To Unsigned Long Integer(number=fpga_settings."Kd_Tau am" ("FPGA Setting")) -> (unsigned 32bit integer=w348:u32)
            n226 = To Unsigned Long Integer(number=fpga_settings."Ki*Tau am" ("FPGA Setting")) -> (unsigned 32bit integer=w346:u32)
            n227 = To Unsigned Long Integer(number=fpga_settings."Kp am" ("FPGA Setting")) -> (unsigned 32bit integer=w351:u32)
            n228 = To Unsigned Long Integer(number=w347) -> (unsigned 32bit integer=w345:u32)
            n229 = To Unsigned Long Integer(number=w350) -> (unsigned 32bit integer=w349:u32)
            n230 = Boolean To (0,1)(Boolean="Feedback AM") -> (0, 1=w358:i16)
            n231 = To Unsigned Long Integer(number=w354) -> (unsigned 32bit integer=w353:u32)
            n232 = To Unsigned Long Integer(number=w358) -> (unsigned 32bit integer=w355:u32)
            n233 = Join Numbers(hi=w346, lo=w345) -> ((hi.lo)=w344:u64)
            n234 = Join Numbers(hi=w348, lo=w349) -> ((hi.lo)=w343:u64)
            n235 = Join Numbers(hi=w351, lo=w353) -> ((hi.lo)=w360:u64)
            n236 = Join Numbers(hi=fpga_settings."Feedback AM" ("FPGA Setting"), lo=w355) -> ((hi.lo)=w356:u64)
            n237 = Build Array(w356, w344, w343, w360) -> (w359:u64[])
            n238 = xnode "Invoke Method"("FPGA VI Reference In"=w361, "Data"=w359) -> ("FPGA VI Reference Out"=w340:T11)  [unwired: 2 in, 2 out]
            n239 = Bundle By Name(cluster=w363, "FPGA ref"=w340) -> (w362:T17)
          }
          event "ch0 DC offset": Value Change {
            n240 = event-data() -> ()  [unwired: 1 in, 6 out]
            n241 = Unbundle By Name(w377) -> ("FPGA ref"=w365:T11)
            n242 = Divide(x=32768, y=5) -> (x/y=w374:dbl)
            n243 = Multiply(x="ch0 DC offset", y=w374) -> (x*y=w373:dbl)
            n244 = Round To Nearest(number=w373) -> (nearest integer value=w372:dbl)
            n245 = To Word Integer(number=w372) -> (16bit integer=w366:i16)
            n246 = xnode "Reinterpret Number"("x"=w366) -> ("y"=w369:fxp<+/-,16,14>)
            n247 = xnode "Reinterpret Number"("x"=w369) -> ("y"=w368:fxp<+,16,16>)
            n248 = call "Write 16bit value.vi"("value"=w368, "FPGA Setting"=fpga_settings."DC_offs 0", "FPGA ref"=w365) -> ("FPGA ref out"=w364:T11)  [unwired: 7 in, 1 out]
            n249 = Bundle By Name(cluster=w377, "FPGA ref"=w364) -> (w376:T17)
          }
          event "Feedback delay", "Trigger delay": Value Change {
            n250 = event-data() -> ()  [unwired: 1 in, 6 out]
            n251 = Add(x="Feedback delay", y="Trigger delay") -> (x+y=w382:u16)
            n252 = xnode "Reinterpret Number"("x"="Trigger delay") -> ("y"=w385:fxp<+/-,16,14>)
            n253 = Unbundle By Name(w391) -> ("FPGA ref"=w386:T11)
            n254 = xnode "Reinterpret Number"("x"=w382) -> ("y"=w389:fxp<+/-,16,14>)
            n255 = xnode "Reinterpret Number"("x"=w385) -> ("y"=w378:fxp<+,16,16>)
            n256 = xnode "Reinterpret Number"("x"=w389) -> ("y"=w388:fxp<+,16,16>)
            n257 = call "Write 16bit value.vi"("value"=w388, "FPGA Setting"=fpga_settings."Feedback delay", "FPGA ref"=w386) -> ("FPGA ref out"=w381:T11)  [unwired: 7 in, 1 out]
            n258 = call "Write 16bit value.vi"("value"=w378, "FPGA Setting"=fpga_settings."Trigger delay", "FPGA ref"=w381) -> ("FPGA ref out"=w380:T11)  [unwired: 7 in, 1 out]
            n259 = Bundle By Name(cluster=w391, "FPGA ref"=w380) -> (w390:T17)
          }
          event "Acquire samples": Value Change {
            n260 = event-data() -> ()  [unwired: 1 in, 6 out]
            n261 = Unbundle By Name(w399) -> ("FPGA ref"=w394:T11)
            n262 = xnode "Reinterpret Number"("x"="Acquire samples") -> ("y"=w397:fxp<+/-,16,14>)
            n263 = xnode "Reinterpret Number"("x"=w397) -> ("y"=w396:fxp<+,16,16>)
            n264 = call "Write 16bit value.vi"("value"=w396, "FPGA Setting"=fpga_settings."Samples to acquire", "FPGA ref"=w394) -> ("FPGA ref out"=w392:T11)  [unwired: 7 in, 1 out]
            n265 = Bundle By Name(cluster=w399, "FPGA ref"=w392) -> (w398:T17)
          }
          event "show setpoint": Value Change {
            n266 = event-data() -> ()  [unwired: 1 in, 6 out]
            n267 = Unbundle By Name(w400) -> ("Feedforward.Setpoint I"=w407:dbl[], "Feedforward.Setpoint Q"=w406:dbl[])
            n268 = Array Size(array=w407) -> (size(s)=w405:i32)
            n269 = Array Size(array=w406) -> (size(s)=w404:i32)
            n270 = Build Array(w407, w406) -> (w408:dbl[][])
            n271 = Greater Than 0?(x=w405) -> (x > 0?=w403:bool)
            n272 = Greater Than 0?(x=w404) -> (x > 0?=w402:bool)
            n273 = And(x=w403, y=w402) -> (x .and. y?=w401:bool)
            n274 = case shown="True" w401 {
              tunnel: w408 -> [_ w409]
              frame False {
              }
              frame True {
                n275 = call "ShowIQvaluesAsync.vi"("IQ data"=w409) -> ()  [unwired: 11 in]
              }
            }
          }
          event "show beam": Value Change {
            n276 = event-data() -> ()  [unwired: 1 in, 6 out]
            n277 = Unbundle By Name(w410) -> ("Feedforward.Beam I"=w417:dbl[], "Feedforward.Beam Q"=w416:dbl[])
            n278 = Array Size(array=w417) -> (size(s)=w415:i32)
            n279 = Array Size(array=w416) -> (size(s)=w414:i32)
            n280 = Build Array(w417, w416) -> (w418:dbl[][])
            n281 = Greater Than 0?(x=w415) -> (x > 0?=w413:bool)
            n282 = Greater Than 0?(x=w414) -> (x > 0?=w412:bool)
            n283 = And(x=w413, y=w412) -> (x .and. y?=w411:bool)
            n284 = case shown="True" w411 {
              tunnel: w418 -> [_ w419]
              frame False {
              }
              frame True {
                n285 = call "ShowIQvaluesAsync.vi"("IQ data"=w419) -> ()  [unwired: 11 in]
              }
            }
          }
          event "show feedforward": Value Change {
            n286 = event-data() -> ()  [unwired: 1 in, 6 out]
            n287 = Unbundle By Name(w420) -> ("Feedforward.Feedforward I"=w427:dbl[], "Feedforward.Feedforward Q"=w426:dbl[])
            n288 = Array Size(array=w427) -> (size(s)=w425:i32)
            n289 = Array Size(array=w426) -> (size(s)=w424:i32)
            n290 = Build Array(w427, w426) -> (w428:dbl[][])
            n291 = Greater Than 0?(x=w425) -> (x > 0?=w423:bool)
            n292 = Greater Than 0?(x=w424) -> (x > 0?=w422:bool)
            n293 = And(x=w423, y=w422) -> (x .and. y?=w421:bool)
            n294 = case shown="True" w421 {
              tunnel: w428 -> [_ w429]
              frame False {
              }
              frame True {
                n295 = call "ShowIQvaluesAsync.vi"("IQ data"=w429) -> ()  [unwired: 11 in]
              }
            }
          }
          event "ch1 DC offset": Value Change {
            n296 = event-data() -> ()  [unwired: 1 in, 6 out]
            n297 = Unbundle By Name(w443) -> ("FPGA ref"=w431:T11)
            n298 = Divide(x=32768, y=5) -> (x/y=w440:dbl)
            n299 = Multiply(x="ch1 DC offset", y=w440) -> (x*y=w439:dbl)
            n300 = Round To Nearest(number=w439) -> (nearest integer value=w438:dbl)
            n301 = To Word Integer(number=w438) -> (16bit integer=w432:i16)
            n302 = xnode "Reinterpret Number"("x"=w432) -> ("y"=w435:fxp<+/-,16,14>)
            n303 = xnode "Reinterpret Number"("x"=w435) -> ("y"=w434:fxp<+,16,16>)
            n304 = call "Write 16bit value.vi"("value"=w434, "FPGA Setting"=fpga_settings."DC_offs 1", "FPGA ref"=w431) -> ("FPGA ref out"=w430:T11)  [unwired: 7 in, 1 out]
            n305 = Bundle By Name(cluster=w443, "FPGA ref"=w430) -> (w442:T17)
          }
          event "Setpoint enabled": Value Change {
            n306 = event-data() -> ()  [unwired: 1 in, 6 out]
            n307 = Unbundle By Name(w453) -> ("FPGA ref"=w447:T11)
            n308 = Boolean To (0,1)(Boolean="Setpoint enabled") -> (0, 1=w444:i16)
            n309 = To Word Integer(number=w444) -> (16bit integer=w448:i16)
            n310 = xnode "Reinterpret Number"("x"=w448) -> ("y"=w451:fxp<+/-,16,14>)
            n311 = xnode "Reinterpret Number"("x"=w451) -> ("y"=w450:fxp<+,16,16>)
            n312 = call "Write 16bit value.vi"("value"=w450, "FPGA Setting"=fpga_settings."Setpoint enable", "FPGA ref"=w447) -> ("FPGA ref out"=w446:T11)  [unwired: 7 in, 1 out]
            n313 = Bundle By Name(cluster=w453, "FPGA ref"=w446) -> (w452:T17)
          }
          event "Beam/FF enabled": Value Change {
            n314 = event-data() -> ()  [unwired: 1 in, 6 out]
            n315 = Unbundle By Name(w463) -> ("FPGA ref"=w457:T11)
            n316 = Boolean To (0,1)(Boolean="Beam/FF enabled") -> (0, 1=w455:i16)
            n317 = To Word Integer(number=w455) -> (16bit integer=w458:i16)
            n318 = xnode "Reinterpret Number"("x"=w458) -> ("y"=w461:fxp<+/-,16,14>)
            n319 = xnode "Reinterpret Number"("x"=w461) -> ("y"=w460:fxp<+,16,16>)
            n320 = call "Write 16bit value.vi"("value"=w460, "FPGA Setting"=fpga_settings."Beam enable", "FPGA ref"=w457) -> ("FPGA ref out"=w456:T11)  [unwired: 7 in, 1 out]
            n321 = Bundle By Name(cluster=w463, "FPGA ref"=w456) -> (w462:T17)
          }
          event Value Change {
            n322 = event-data() -> ()  [unwired: 1 in, 6 out]
            n323 = Unbundle By Name(w467) -> ("FPGA ref"=w469:T11)
            n324 = property on="Rumode" class="Bool (strict)"("Val(Sgnl)"=FALSE ("Value (Signaling)")) -> ()  [unwired: 2 in, 2 out]
            n325 = xnode "Read/Write Control"("FPGA VI Reference In"=w469, "Mode"="Mode") -> ("FPGA VI Reference Out"=w468:T11)  [unwired: 1 in, 1 out]
            n326 = Bundle By Name(cluster=w467, "FPGA ref"=w468, "data mode"="Mode") -> (w466:T17)
          }
          event Value Change {
            n327 = event-data() -> ()  [unwired: 1 in, 6 out]
            n328 = Bundle By Name(cluster=w471, "5782 Trigger"="Trigger") -> (w470:T17)
          }
          event "High speed transfer to host": Value Change {
            w475 = dbl[][] [] ("History Data")
            n329 = event-data() -> ()  [unwired: 1 in, 3 out]
            n330 = Multiply(x=10, y=w491) -> (x*y=w489:i32)
            n331 = Select(t=w489, s="High speed transfer to host", f=w491) -> (s? t:f=w477:i32)
            n332 = Unbundle By Name(w486) -> ("FPGA ref"=w484:T11)
            n333 = Select(t=0.0001, s="High speed transfer to host", f=0.001 ("t")) -> (s? t:f=w482:dbl)
            n334 = property on="Lower chart" class="WFChart (strict)"("History Data"=w475) -> ()  [unwired: 2 in, 2 out]
            n335 = Dynamic FPGA Interface Cast(Session In=w488, Type=w484) -> (Session Out=w487:refnum<k20>)
            n336 = property on="Upper chart" class="WFChart (strict)"("History Data"=w475) -> (error out=w476:errorcluster)  [unwired: 2 in, 1 out]
            n337 = Initialize Array(nan ("element"), 4 ("dimension size"), w477) -> (w479:dbl[][])
            n338 = xnode "Read/Write Control"("FPGA VI Reference In"=w487, "5782 record length"=w477, "Full speed transfer"="High speed transfer to host") -> ()  [unwired: 1 in, 2 out]
            n339 = property on="Upper chart" class="WFChart (strict)"("XScale.Multiplier"=w482) -> ()  [unwired: 2 in, 2 out]
            n340 = flat-sequence {
              tunnel: w479 -> [w493]
              tunnel: [w492] -> w474
              tunnel: w476 -> [_]
              frame #0 {
                n341 = local write "Upper chart"(w493) -> ()
                n342 = local read "Zoom time X"() -> (w492:bool)
              }
            }
            n343 = Bundle By Name(cluster=w486, "FPGA ref"=w484, "samples per record"=w477) -> (w485:T17)
            n344 = property on="Zoom time X" class="Bool (strict)"("Val(Sgnl)"=w474) -> ()  [unwired: 2 in, 2 out]
          }
          event "Samples per 5782 record": Value Change {
            n345 = event-data() -> ()  [unwired: 1 in, 6 out]
            n346 = Unbundle By Name(w495) -> ("FPGA ref"=w498:T11)
            n347 = xnode "Read/Write Control"("FPGA VI Reference In"=w498, "5782 record length"="Samples per 5782 record") -> ("FPGA VI Reference Out"=w497:T11)  [unwired: 1 in, 1 out]
            n348 = Bundle By Name(cluster=w495, "FPGA ref"=w497, "samples per record"="Samples per 5782 record") -> (w494:T17)
          }
          event "Singleshot": Value Change {
            n349 = event-data() -> ()  [unwired: 1 in, 6 out]
            n350 = local write "Rumode"(FALSE ("Rumode")) -> ()
            n351 = Bundle By Name(cluster=w505, "scope mode"=ScopeMode."Single") -> (w500:T17)
            n352 = call "ToggleContinousMode.vi"("Cont Acquisition"=FALSE, "scope in"=w500) -> ("scope out"=w499:T17)  [unwired: 8 in, 1 out]
            n353 = call "ToggleAqcuisitionRunning_5782.vi"("Acquisition running"=TRUE, "scope in"=w499) -> ("scope out"=w503:T17)  [unwired: 8 in, 1 out]
            n354 = call "SendSWtrigger_5782.vi"("scope in"=w503) -> ("scope out"=w502:T17)  [unwired: 9 in, 1 out]
          }
          event "Rumode": Value Change {
            n355 = event-data() -> ()  [unwired: 1 in, 6 out]
            n356 = case shown="\"Triggered\"" "Trigmode" {
              tunnel: [ScopeMode."Running" ("scope mode") ScopeMode."Continuous" ("scope mode")] -> w508
              frame "Triggered" {
              }
              frame "Continuous" {
              }
            }
            n357 = Select(t=w508, s="Rumode", f=ScopeMode."Stopped" ("scope mode")) -> (s? t:f=w512:T18)
            n358 = Bundle By Name(cluster=w513, "scope mode"=w512) -> (w511:T17)
            n359 = case shown="\"Single\", \"Running\"" w512 {
              tunnel: w511 -> [w520 w527 w531]
              tunnel: [w521 w525 w532] -> w510
              frame "Single", "Running" {
                n360 = call "ToggleContinousMode.vi"("Cont Acquisition"=FALSE, "scope in"=w520) -> ("scope out"=w518:T17)  [unwired: 8 in, 1 out]
                n361 = call "ToggleAqcuisitionRunning_5782.vi"("Acquisition running"=TRUE, "scope in"=w518) -> ("scope out"=w522:T17)  [unwired: 8 in, 1 out]
                n362 = call "SendSWtrigger_5782.vi"("scope in"=w522) -> ("scope out"=w521:T17)  [unwired: 9 in, 1 out]
              }
              frame "Continuous" {
                n363 = call "ToggleAqcuisitionRunning_5782.vi"("Acquisition running"=TRUE, "scope in"=w527) -> ("scope out"=w526:T17)  [unwired: 8 in, 1 out]
                n364 = call "ToggleContinousMode.vi"("Cont Acquisition"=TRUE ("Acquisition running"), "scope in"=w526) -> ("scope out"=w525:T17)  [unwired: 8 in, 1 out]
              }
              frame "Stopped" {
                n365 = call "ToggleContinousMode.vi"("Cont Acquisition"=FALSE, "scope in"=w531) -> ("scope out"=w529:T17)  [unwired: 8 in, 1 out]
                n366 = call "ToggleAqcuisitionRunning_5782.vi"("Acquisition running"=FALSE, "scope in"=w529) -> ("scope out"=w532:T17)  [unwired: 8 in, 1 out]
              }
            }
          }
          event Value Change {
            n367 = event-data() -> ("CtlRef"=w536:refnum<vi>, "NewVal"=w534:bool)  [unwired: 1 in, 4 out]
            n368 = Search 1D Array(1D array=w537, element=w536) -> (index of element=w535:i32)  [unwired: 1 in]
            n369 = property on="Upper graph" class="WFGraph (strict)"("Active Plot"=w535, "Plot.Visible?"=w534) -> ()  [unwired: 2 in, 2 out]
            n370 = property on="Upper chart" class="WFChart (strict)"("Active Plot"=w535, "Plot.Visible?"=w534) -> ()  [unwired: 2 in, 2 out]
          }
          event Value Change {
            n371 = event-data() -> ("CtlRef"=w548:refnum<vi>, "NewVal"=w540:bool)  [unwired: 1 in, 4 out]
            n372 = local read "unwrap phase"() -> (w542:bool)
            n373 = Search 1D Array(1D array=w547, element=w548) -> (index of element=w546:i32)  [unwired: 1 in]
            n374 = Add(x=w546, y=2) -> (x+y=w544:i32)
            n375 = property on="freqdata" class="WFGraph (strict)"("Active Plot"=w546, "Plot.Visible?"=w540) -> ()  [unwired: 2 in, 2 out]
            n376 = Not(x=w542) -> (.not. x?=w541:bool)
            n377 = And(x=w542, y=w540) -> (x .and. y?=w543:bool)
            n378 = And(x=w541, y=w540) -> (x .and. y?=w539:bool)
            n379 = property on="Lower chart" class="WFChart (strict)"("Active Plot"=w546, "Plot.Visible?"=w539, "Active Plot"=w544, "Plot.Visible?"=w543) -> ()  [unwired: 2 in, 2 out]
          }
          event "unwrap phase": Value Change {
            n380 = event-data() -> ()  [unwired: 1 in, 6 out]
            n381 = local read "Ch0"() -> (w552:bool)
            n382 = local read "Ch1"() -> (w554:bool)
            n383 = Not(x="unwrap phase") -> (.not. x?=w557:bool)
            n384 = And(x=w552, y=w557) -> (x .and. y?=w556:bool)
            n385 = And(x=w554, y=w557) -> (x .and. y?=w555:bool)
            n386 = And(x=w554, y="unwrap phase") -> (x .and. y?=w553:bool)
            n387 = And(x=w552, y="unwrap phase") -> (x .and. y?=w550:bool)
            n388 = property on="Lower chart" class="WFChart (strict)"("Active Plot"=u32 0, "Plot.Visible?"=w556, "Active Plot"=u32 1, "Plot.Visible?"=w555) -> ()  [unwired: 2 in, 2 out]
            n389 = property on="Lower chart" class="WFChart (strict)"("Active Plot"=u32 2, "Plot.Visible?"=w553, "Active Plot"=u32 3, "Plot.Visible?"=w550) -> ()  [unwired: 2 in, 2 out]
          }
          event User Event {
            n390 = event-data() -> ("Sender"=w565:string, "Variant"=w564:variant, "driver status"=w563:T14)  [unwired: 1 in, 5 out]
            n391 = Unbundle By Name(w567) -> ("RemoteConnection"=w569:refnum<class "RemoteConnection.lvclass">)
            n392 = call "HandleRemoteMessage.vi"("driver status"=w563, "Message data"=w564, "Sender"=w565, "RemoteConnection in"=w569) -> ("RemoteConnection out"=w568:refnum<class "RemoteConnection.lvclass">)  [unwired: 6 in, 1 out]
            n393 = Bundle By Name(cluster=w567, "RemoteConnection"=w568) -> (w566:T17)
          }
          event "stop": Value Change {
            n394 = event-data() -> ()  [unwired: 1 in, 6 out]
          }
          event Value Change {
            n395 = event-data() -> ()  [unwired: 1 in, 6 out]
            n396 = case shown="\"V\"" "Unit" {
              tunnel: ["V" "dBV" "V^2"] -> w574
              frame "V" {
              }
              frame "dBV" {
              }
              frame "V^2" {
              }
            }
            n397 = Concatenate Strings("Amplitude [", w574, "]") -> (w572:string)
            n398 = property on="freqdata" class="WFGraph (strict)"("YScale.NameLbl.Text"=w572) -> ()  [unwired: 2 in, 2 out]
          }
          event "#bins": Value Change {
            n399 = event-data() -> ()  [unwired: 1 in, 6 out]
            n400 = local read "Upper chart"() -> (w583:dbl[][])
            n401 = local read "Window"() -> (w584:T4)
            n402 = local read "Unit"() -> (w585:T3)
            n403 = call "calc FFT.vi"("#bins"="#bins", "dt"=1e-06, "Unit"=w585, "Window"=w584, "data"=w583) -> ("Power Spectrum / PSD"=w582:cluster{"f0":dbl, "df":dbl, "magnitude":dbl[]}[])  [unwired: 6 in]
            n404 = local write "freqdata"(w582) -> ()
          }
          event "Zoom time X", "Zoom time Y": Value Change {
            n405 = event-data() -> ()  [unwired: 1 in, 6 out]
            n406 = control-ref of="Upper chart"() -> (w590:refnum<vi>)
            n407 = control-ref of="Upper graph"() -> (w591:refnum<vi>)
            n408 = call "setZoomTool.vi"("Zoom Y"="Zoom time Y", "Zoom  X"="Zoom time X", "reference"=w590) -> ()  [unwired: 9 in]
            n409 = call "setZoomTool.vi"("Zoom Y"="Zoom time Y", "Zoom  X"="Zoom time X", "reference"=w591) -> ()  [unwired: 9 in]
          }
          event "Zoom freq Y", "Zoom freq X": Value Change {
            n410 = event-data() -> ()  [unwired: 1 in, 6 out]
            n411 = control-ref of="Lower chart"() -> (w596:refnum<vi>)
            n412 = control-ref of="Lower graph"() -> (w595:refnum<vi>)
            n413 = control-ref of="freqdata"() -> (w597:refnum<vi>)
            n414 = call "setZoomTool.vi"("Zoom Y"="Zoom freq Y", "Zoom  X"="Zoom freq X", "reference"=w597) -> ()  [unwired: 9 in]
            n415 = call "setZoomTool.vi"("Zoom Y"="Zoom freq Y", "Zoom  X"="Zoom freq X", "reference"=w596) -> ()  [unwired: 9 in]
            n416 = call "setZoomTool.vi"("Zoom Y"="Zoom freq Y", "Zoom  X"="Zoom freq X", "reference"=w595) -> ()  [unwired: 9 in]
          }
          event Value Change {
            w601 = dbl[][] [] ("History Data")
            n417 = event-data() -> ()  [unwired: 1 in, 6 out]
            n418 = property on="Upper chart" class="WFChart (strict)"("History Data"=w601) -> ()  [unwired: 2 in, 2 out]
            n419 = property on="Lower chart" class="WFChart (strict)"("History Data"=w601) -> ()  [unwired: 2 in, 2 out]
            n420 = local write "freqdata"(cluster{"f0":dbl, "df":dbl, "magnitude":dbl[]}[] [] ("freqdata")) -> ()
            n421 = call "UpdateGraphs.vi"("Buffer mode"="Buffer", "Display mode"="Display", "Graph_refs"=w602) -> ()  [unwired: 9 in]
            n422 = property on="Zoom time X" class="Bool (strict)"("Val(Sgnl)"=TRUE ("Value (Signaling)")) -> ()  [unwired: 2 in, 2 out]
          }
          event "Feed forward": Value Change {
            n423 = event-data() -> ()  [unwired: 1 in, 6 out]
            n424 = control-ref of="show feedforward"() -> (w609:refnum<vi>)
            n425 = call "LoadFeedforward.vi"("show ref"=w609, "Path"="Feed forward") -> ("error out"=w610:errorcluster, "values Q"=w613:dbl[], "values I"=w612:dbl[])  [unwired: 7 in]
            n426 = case shown="No Error" w610 {
              tunnel: w614 -> [w621 w624]
              tunnel: w613 -> [w622 _]
              tunnel: w612 -> [w623 _]
              tunnel: [w615 w624] -> w611
              tunnel: w608 -> [w619 _]
              tunnel: Memory_block."Beam" ("Memory block") -> [w620 _]
              frame No Error {
                n427 = Bundle By Name(cluster=w621, "Feedforward.Feedforward I"=w623, "Feedforward.Feedforward Q"=w622) -> (w618:T17)
                n428 = call "GetFeedforward.vi"("scope in"=w618) -> ("values Q"=w616:dbl[], "values I"=w617:dbl[], "scope out"=w615:T17)  [unwired: 8 in]
                n429 = call "WriteFeedForward.vi"("Memory block"=w620, "values Q"=w616, "values I"=w617, "FPGA VI Reference"=w619) -> ()  [unwired: 7 in, 1 out]
              }
              frame Error {
              }
            }
          }
          event "Beam": Value Change {
            n430 = event-data() -> ()  [unwired: 1 in, 6 out]
            n431 = control-ref of="show beam"() -> (w628:refnum<vi>)
            n432 = call "LoadFeedforward.vi"("show ref"=w628, "Path"="Beam") -> ("error out"=w629:errorcluster, "values Q"=w632:dbl[], "values I"=w631:dbl[])  [unwired: 7 in]
            n433 = case shown="No Error" w629 {
              tunnel: w633 -> [w640 w643]
              tunnel: w632 -> [w641 _]
              tunnel: w631 -> [w642 _]
              tunnel: [w634 w643] -> w630
              tunnel: w627 -> [w638 _]
              tunnel: Memory_block."Beam" ("Memory block") -> [w639 _]
              frame No Error {
                n434 = Bundle By Name(cluster=w640, "Feedforward.Beam I"=w642, "Feedforward.Beam Q"=w641) -> (w637:T17)
                n435 = call "GetFeedforward.vi"("scope in"=w637) -> ("values Q"=w635:dbl[], "values I"=w636:dbl[], "scope out"=w634:T17)  [unwired: 8 in]
                n436 = call "WriteFeedForward.vi"("Memory block"=w639, "values Q"=w635, "values I"=w636, "FPGA VI Reference"=w638) -> ()  [unwired: 7 in, 1 out]
              }
              frame Error {
              }
            }
          }
          event "Setpoint": Value Change {
            n437 = event-data() -> ()  [unwired: 1 in, 6 out]
            n438 = control-ref of="show setpoint"() -> (w647:refnum<vi>)
            n439 = call "LoadFeedforward.vi"("show ref"=w647, "Path"="Setpoint") -> ("error out"=w648:errorcluster, "values Q"=w651:dbl[], "values I"=w650:dbl[])  [unwired: 7 in]
            n440 = case shown="No Error" w648 {
              tunnel: w652 -> [w658 w659]
              tunnel: w651 -> [w654 _]
              tunnel: w650 -> [w655 _]
              tunnel: [w653 w659] -> w649
              tunnel: w646 -> [w656 _]
              tunnel: Memory_block."Setpoint" ("Memory block") -> [w657 _]
              frame No Error {
                n441 = call "WriteFeedForward.vi"("Memory block"=w657, "values Q"=w654, "values I"=w655, "FPGA VI Reference"=w656) -> ()  [unwired: 7 in, 1 out]
                n442 = Bundle By Name(cluster=w658, "Feedforward.Setpoint I"=w655, "Feedforward.Setpoint Q"=w654) -> (w653:T17)
              }
              frame Error {
              }
            }
          }
        }
      }
      "stop 2" <- w126
    }
    frame Error {
    }
  }
  n443 = Unregister For Events(event registration refnum=w81) -> ()  [unwired: 1 in, 1 out]
  n444 = Unbundle By Name(w64) -> ("FPGA ref"=w88:T11, "RemoteConnection"=w26:refnum<class "RemoteConnection.lvclass">)
  n445 = flat-sequence {
    tunnel: w88 -> [w664]
    tunnel: w26 -> [w663]
    frame #0 {
      n446 = call "Close.vi"("RemoteConnection in"=w663) -> ()  [unwired: 9 in, 2 out]
      n447 = xnode "Close FPGA VI Reference"("FPGA VI Reference In"=w664) -> ()  [unwired: 1 in, 1 out]
      n448 = global write "global_stop.vi" "Stop"(TRUE ("Stop")) -> ()
    }
  }
